vi "PushCycle.vi"(4 "maxVolume_uL":dbl, 5 "DispenseAnalyte":string, 9 "speed_uL_s":dbl, 10 "volume_uL":dbl, 11 "Pump_Refnum":refnum<k24>) -> (3 "Pump":refnum<k24>)   [LabVIEW 2020]
uses:
  C:/Users/bashc/Desktop/ChannelAutomatorR_.06/PumpAdapter.exe
  PumpAdapter.exe
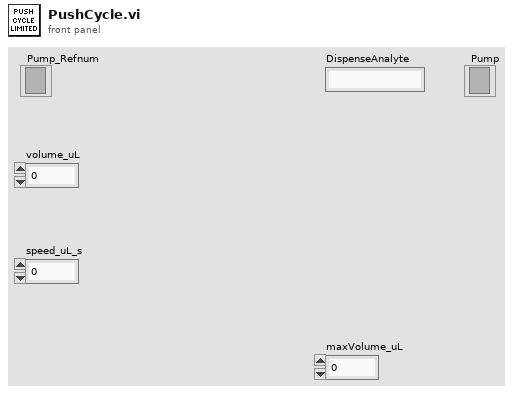
[diagram p1: front panel]
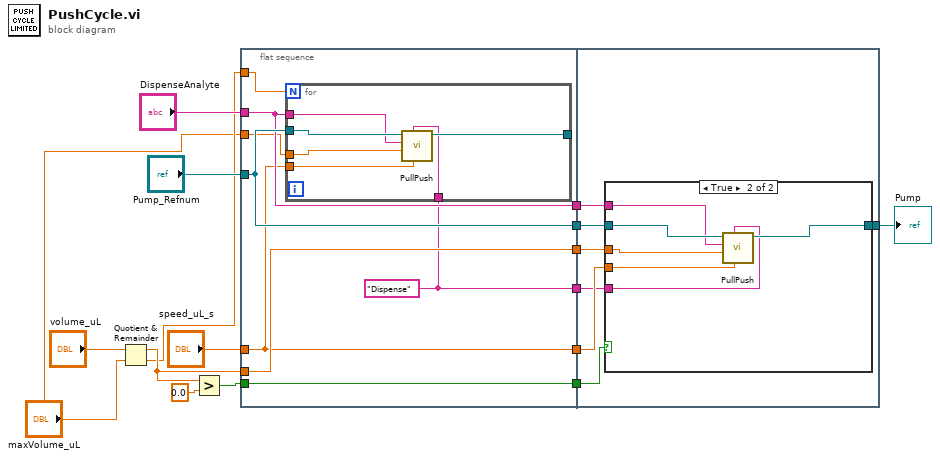
[diagram p0: block diagram]
diagram:
  n1 = Quotient & Remainder(x="volume_uL", y="maxVolume_uL") -> (x-y*floor(x/y)=w12:dbl, floor(x/y)=w3:dbl)
  n2 = Greater?(x=w12, y=0.0) -> (0:w16:bool)
  n3 = flat-sequence {
    tunnel: "DispenseAnalyte" -> [w20]
    tunnel: "Pump_Refnum" -> [w21]
    tunnel: w12 -> [w23]
    tunnel: "speed_uL_s" -> [w19]
    tunnel: w16 -> [w24]
    tunnel: [w24] -> w8
    tunnel: [w19] -> w7
    tunnel: [w23] -> w6
    tunnel: [w21] -> w5
    tunnel: [w20] -> w4
    tunnel: w3 -> [w22]
    tunnel: "maxVolume_uL" -> [w18]
    tunnel: [w17] -> w1
    tunnel: [w32] -> w9
    tunnel: w8 -> [w37]
    tunnel: w7 -> [w36]
    tunnel: w6 -> [w35]
    tunnel: w5 -> [w34]
    tunnel: w4 -> [w33]
    tunnel: w1 -> [w31]
    frame #0 {
      w17 = "Dispense" ("pushTo")
      n4 = for {
        N: w22 -> [_]
        tunnel: w21 -> [w30]
        tunnel: w20 -> [w26]
        tunnel: w19 -> [w29]
        tunnel: w18 -> [w27]
        tunnel: [w28] -> _
        tunnel: w17 -> [w25]
        n5 = call "PullPush.vi"("speed_uL_s"=w29, "pushTo"=w25, "volume_uL"=w27, "pullFrom"=w26, ".NET Refnum in"=w30) -> (".NET Refnum out"=w28:refnum<k24>)  [unwired: 6 in]
      }
    }
    frame #1 {
      n6 = case shown="True" w37 {
        tunnel: w35 -> [_ w43]
        tunnel: [w38 w44] -> w32
        tunnel: w34 -> [w38 w41]
        tunnel: w36 -> [_ w42]
        tunnel: w33 -> [_ w40]
        tunnel: w31 -> [_ w39]
        frame False {
        }
        frame True {
          n7 = call "PullPush.vi"("speed_uL_s"=w42, "pushTo"=w39, "volume_uL"=w43, "pullFrom"=w40, ".NET Refnum in"=w41) -> (".NET Refnum out"=w44:refnum<k24>)  [unwired: 6 in]
        }
      }
    }
  }
  "Pump" <- w9
